vi "Intensity Graph Linecut (Vertical) (by ref).vi"(6 "Averaging Method":enum16{"Step", "Gaussian"}(ring), 8 "error in (no error)":errorcluster, 9 "width (vertical)":dbl, 11 "graph_utilities in":refnum<class "graph_utilities.lvclass">) -> (0 "error out":errorcluster, 3 "graph_utilities out":refnum<class "graph_utilities.lvclass">)   [LabVIEW 2019, in "graph_utilities.lvclass"]
doc: "Takes a Vertical Linecut of an Intensity Graph and outputs to an XY Graph. The center location of the linecut is determined by the x-position of the Intensity Graph's curser.\n - <b>width</b> is the standard deviation of a Gaussian function in the units of the Intensity Graph x scale.\n - If <b>width = 0 </b> the spacing between two adjacent data points will be used."
uses:
  graph_utilities.lvclass
  <vilib>/Analysis/baseanly.llb/A x Vector.vi
  <vilib>/Analysis/NI_AALBase.lvlib
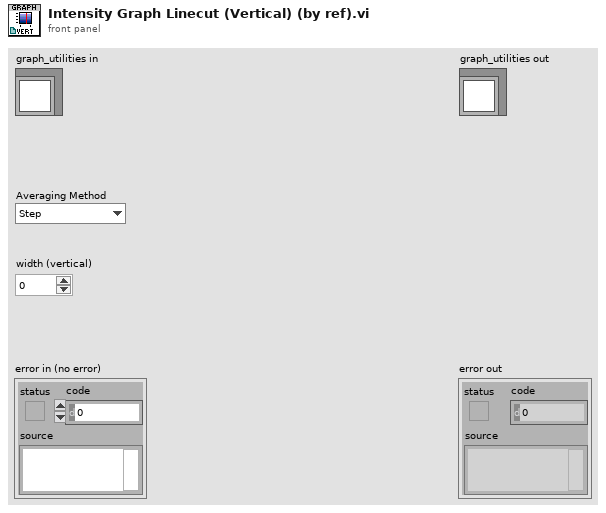
[diagram p1: front panel]
types:
  T1 = typedef "LVPointDoubleTypeDef.ctl" = cluster{"X":dbl, "Y":dbl}
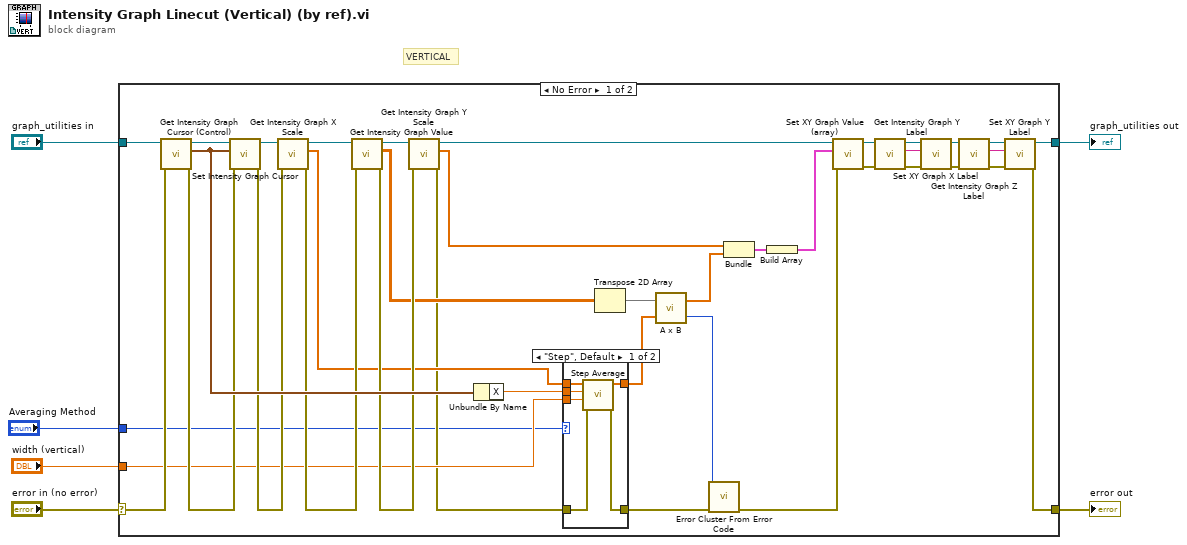
[diagram p0: block diagram]
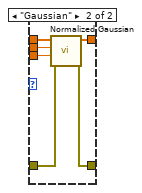
[diagram p2: hidden frame]
diagram:
  # "VERTICAL"
  n1 = case shown="No Error" "error in (no error)" {
    selector: "error in (no error)" -> [w38 w59]
    tunnel: [w9 w59] -> w5
    tunnel: [w8 w58] -> w3
    tunnel: "graph_utilities in" -> [w41 w58]
    tunnel: "width (vertical)" -> [w27 _]
    tunnel: "Averaging Method" -> [w7 _]
    frame No Error {
      n2 = call "Get Intensity Graph Cursor (Control).vi"("error in (no error)"=w38, "graph_utilities in"=w41) -> ("error out"=w37:errorcluster, "Cursor.Cursor Position"=w39:T1, "graph_utilities out"=w42:refnum<class "graph_utilities.lvclass">)  [unwired: 7 in]
      n3 = call "Set Intensity Graph Cursor.vi"("error in (no error)"=w37, "Cursor.Cursor Position"=w39, "graph_utilities in"=w42) -> ("error out"=w36:errorcluster, "graph_utilities out"=w40:refnum<class "graph_utilities.lvclass">)  [unwired: 7 in]
      n4 = call "Get Intensity Graph X Scale.vi"("error in (no error)"=w36, "graph_utilities in"=w40) -> ("error out"=w33:errorcluster, "X Scale"=w29:dbl[], "graph_utilities out"=w35:refnum<class "graph_utilities.lvclass">)  [unwired: 6 in, 1 out]
      n5 = call "Get Intensity Graph Value.vi"("error in (no error)"=w33, "graph_utilities in"=w35) -> ("error out"=w32:errorcluster, "Value"=w31:dbl[][], "graph_utilities out"=w34:refnum<class "graph_utilities.lvclass">)  [unwired: 7 in]
      n6 = call "Get Intensity Graph Y Scale.vi"("error in (no error)"=w32, "graph_utilities in"=w34) -> ("error out"=w25:errorcluster, "Y Scale"=w30:dbl[], "graph_utilities out"=w22:refnum<class "graph_utilities.lvclass">)  [unwired: 6 in, 1 out]
      n7 = Unbundle By Name(w39) -> ("X"=w28:dbl)
      n8 = case shown="\"Step\", Default" w7 {
        tunnel: w29 -> [w51 w57]
        tunnel: w28 -> [w50 w56]
        tunnel: w27 -> [w49 w55]
        tunnel: [w47 w54] -> w26
        tunnel: w25 -> [w48 w53]
        tunnel: [w46 w52] -> w24
        frame "Step", Default {
          n9 = call "Step Average.vi"("error in (no error)"=w48, "width (c)"=w49, "position (b)"=w50, "Scale"=w51) -> ("error out"=w46:errorcluster, "Averaged Result"=w47:dbl[])  [unwired: 4 in, 2 out]
        }
        frame "Gaussian" {
          n10 = call "Normalized Gaussian.vi"("error in (no error)"=w53, "width (c)"=w55, "position (b)"=w56, "Scale"=w57) -> ("error out"=w52:errorcluster, "Normalized Gaussian"=w54:dbl[])  [unwired: 6 in]
        }
      }
      n11 = Transpose 2D Array(2D array=w31) -> (transposed array=w45:dbl[][])
      n12 = call-poly <vilib>:"A x B.vi"("Vector"=w26, "A"=w45) -> ("error"=w43:i32, "A x Vector"=w44:dbl[])
      n13 = call <vilib>:"Error Cluster From Error Code.vi"("error in (no error)"=w24, "error code (0)"=w43) -> ("error out"=w21:errorcluster)  [unwired: 7 in]
      n14 = Bundle("Y Scale"=w30, "A x Vector"=w44) -> (w23:cluster{"Y Scale":dbl[], "A x Vector":dbl[]})  [unwired: 1 in]
      n15 = Build Array(w23) -> (w20:cluster{"Y Scale":dbl[], "A x Vector":dbl[]}[])
      n16 = call "Set XY Graph Value (array).vi"("error in (no error)"=w21, "XY-data"=w20, "graph_utilities in"=w22) -> ("error out"=w10:errorcluster, "graph_utilities out"=w15:refnum<class "graph_utilities.lvclass">)  [unwired: 7 in]
      n17 = call "Get Intensity Graph Y Label.vi"("error in (no error)"=w10, "graph_utilities in"=w15) -> ("error out"=w13:errorcluster, "Y Label"=w16:string, "graph_utilities out"=w14:refnum<class "graph_utilities.lvclass">)  [unwired: 7 in]
      n18 = call "Set XY Graph X Label.vi"("error in (no error)"=w13, "X Label"=w16, "graph_utilities in"=w14) -> ("error out"=w11:errorcluster, "graph_utilities out"=w12:refnum<class "graph_utilities.lvclass">)  [unwired: 7 in]
      n19 = call "Get Intensity Graph Z Label.vi"("error in (no error)"=w11, "graph_utilities in"=w12) -> ("error out"=w17:errorcluster, "Z Label"=w19:string, "graph_utilities out"=w18:refnum<class "graph_utilities.lvclass">)  [unwired: 7 in]
      n20 = call "Set XY Graph Y Label.vi"("error in (no error)"=w17, "Y Label"=w19, "graph_utilities in"=w18) -> ("error out"=w9:errorcluster, "graph_utilities out"=w8:refnum<class "graph_utilities.lvclass">)  [unwired: 7 in]
    }
    frame Error {
    }
  }
  "error out" <- w5
  "graph_utilities out" <- w3
